vi "Enable PRBS.vi"(8 "error in (no error)":errorcluster, 10 "Enable PRBS (Disabled)":bool, 11 "VISA resource name":refnum<visa-resource-name>) -> (0 "error out":errorcluster, 3 "VISA resource name out":refnum<visa-resource-name>)   [LabVIEW 2013, in "Stanford Research CG635.lvlib"]
doc: "<b>Enable</b> or <b>disable</b> the Pseudorandom binary sequence.\n\nDefault: Disabled"
uses:
  <instrlib>/Stanford Research CG635/Stanford Research CG635.lvlib
panel:
  # "Enabled"
  # "Disabled"
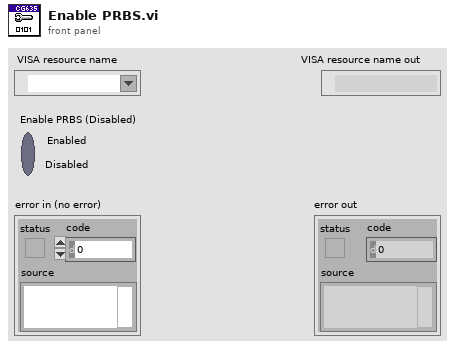
[diagram p1: front panel]
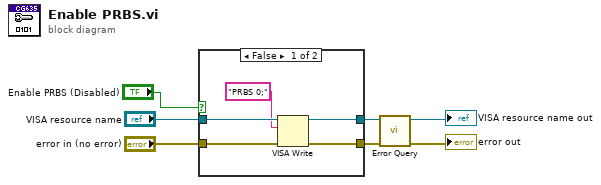
[diagram p0: block diagram]
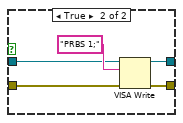
[diagram p2: hidden frame]
diagram:
  n1 = case shown="False" "Enable PRBS (Disabled)" {
    tunnel: [w10 w16] -> w7
    tunnel: [w9 w15] -> w6
    tunnel: "VISA resource name" -> [w12 w14]
    tunnel: "error in (no error)" -> [w11 w13]
    frame False {
      n2 = VISA Write(VISA resource name=w12, write buffer="PRBS 0;", error in (no error)=w11) -> (VISA resource name out=w10:refnum<visa-resource-name>, error out=w9:errorcluster)  [unwired: 1 out]
    }
    frame True {
      n3 = VISA Write(VISA resource name=w14, write buffer="PRBS 1;", error in (no error)=w13) -> (VISA resource name out=w16:refnum<visa-resource-name>, error out=w15:errorcluster)  [unwired: 1 out]
    }
  }
  n4 = call <instrlib>:"Error Query.vi"("error in (no error)"=w6, "VISA resource name"=w7) -> ("error out"=→"error out":errorcluster, "VISA resource name out"=→"VISA resource name out":refnum<visa-resource-name>)  [unwired: 6 in, 2 out]
